vi "CreateCANReadQueues.vi"(11 "Queues":refnum<queue>) -> (0 "error out":errorcluster, 2 "timed out?":bool, 3 "CAN frame":T1 {"type" items=["CAN Data", "CAN Remote"]; "identifier" format="%.0x"})   [LabVIEW 2016, in "DSI-RT.lvlib"]
uses:
  DSI-RT.lvlib
  <vilib>/RioEmbeddedCAN/RioEmbeddedCAN.llb/CANFrameControl.ctl
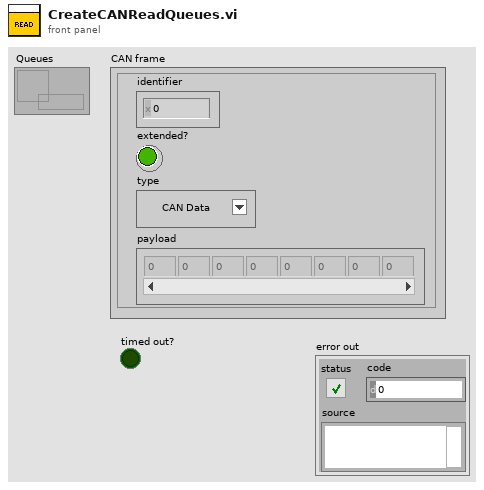
[diagram p1: front panel]
types:
  T1 = typedef "CANFrameControl.ctl" = cluster{"identifier":u32, "extended?":bool, "type":u8, "payload":u8[]}
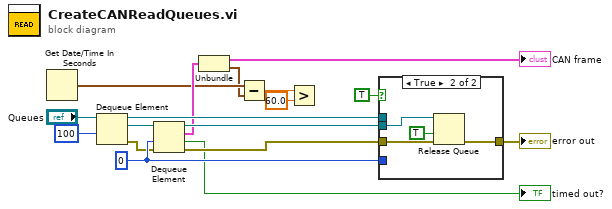
[diagram p0: block diagram]
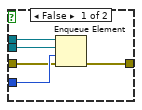
[diagram p2: hidden frame]
diagram:
  w17 = 0 ("timeout in ms (-1)")
  n1 = Get Date/Time In Seconds() -> (seconds since 1Jan1904=w5:timestamp)
  n2 = Dequeue Element(queue="Queues", timeout in ms (-1)=100) -> (queue out=w14:refnum<queue>, element=w12:refnum<queue>, error out=w13:errorcluster)  [unwired: 1 in, 1 out]
  n3 = Dequeue Element(queue=w12, timeout in ms (-1)=w17, error in (no error)=w13) -> (queue out=w15:refnum<queue>, element=w10:cluster{"CAN frame":T1, "Timestamp":timestamp}, timed out?=→"timed out?":bool, error out=w16:errorcluster)
  n4 = Unbundle(w10) -> ("CAN frame"=→"CAN frame":T1, "Timestamp"=w4:timestamp)
  n5 = Subtract(x=w5, y=w4) -> (x-y=w3:dbl)
  n6 = Greater?(x=w3, y=60.0) -> ()  [unwired: 1 out]
  n7 = case shown="True" TRUE {
    tunnel: w17 -> [w22 _]
    tunnel: w16 -> [w21 w26]
    tunnel: [w20 w25] -> w8
    tunnel: w15 -> [w19 w24]
    tunnel: w14 -> [w18 _]
    frame False {
      n8 = Enqueue Element(queue=w18, element=w19, timeout in ms (-1)=w22, error in (no error)=w21) -> (error out=w20:errorcluster)  [unwired: 2 out]
    }
    frame True {
      n9 = Release Queue(queue=w24, force destroy? (F)=TRUE, error in (no error)=w26) -> (error out=w25:errorcluster)  [unwired: 2 out]
    }
  }
  "error out" <- w8
